vi "VA CoAP - Message - DECODE.vi"(0 "CoAP Message":string) -> (4 "CoAP Message Decoded":T1 {"Type" items=["CONfimable", "NON-confirmable", "ACKnowledgement", "ReSeT"]}, 8 "CoAP Message":u8[](array[numeric]), 10 "Valid?":bool, 15 "Format Error?":bool)   [LabVIEW 2020]
uses:
  data types/VA CoAP - Message.ctl
  data types/VA CoAP - Message - Type.ctl
  data types/VA CoAP - Message - Options.ctl
  data types/VA CoAP - Message - Options - 11 Uri-Path.ctl
panel:
  out "Paths":string[](array[string])
  out "Token Length":u8
  out "2nd LSB is 1?":bool
  out "1st LSB is 0?":bool
  out "Ate least 4 Bytes?":bool
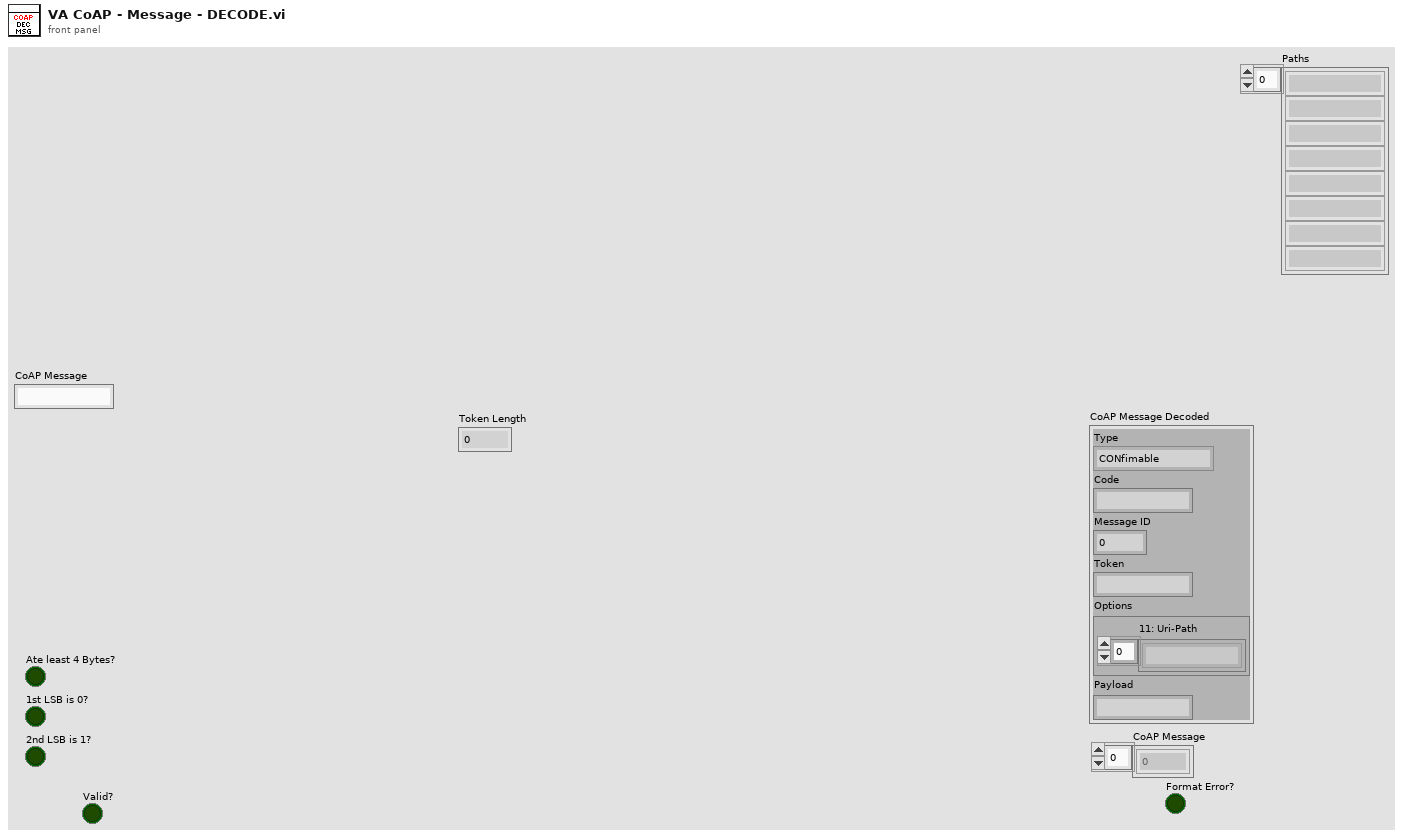
[diagram p1: front panel]
types:
  T1 = typedef "VA CoAP - Message.ctl" = cluster{"Type":T2, "Code":string, "Message ID":u16, "Token":string, "Options":T3, "Payload":string}
  T2 = typedef "VA CoAP - Message - Type.ctl" = u8
  T3 = typedef "VA CoAP - Message - Options.ctl" = cluster{"11: Uri-Path":T4}
  T4 = typedef "VA CoAP - Message - Options - 11 Uri-Path.ctl" = string[]
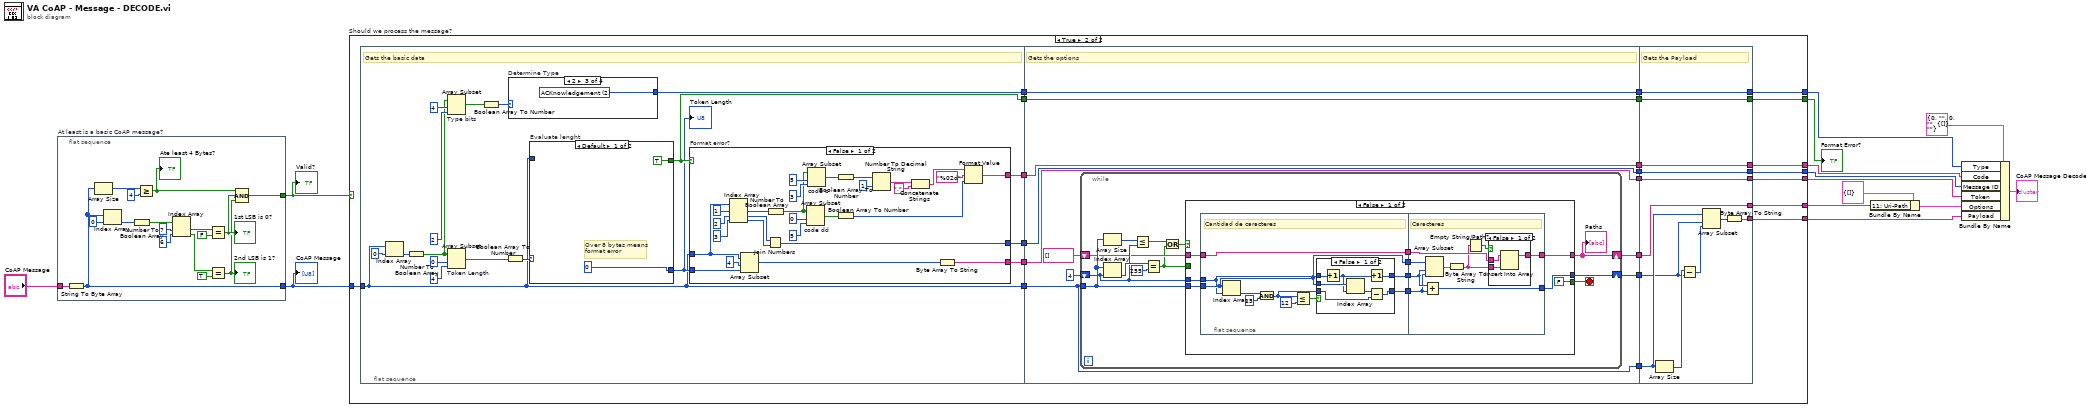
[diagram p0: block diagram]
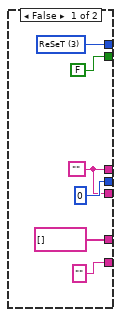
[diagram p2: hidden frame]
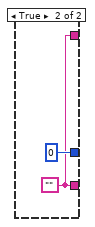
[diagram p3: hidden frame]
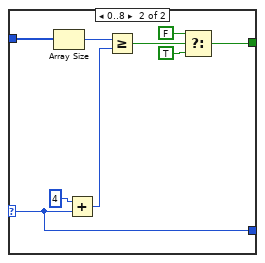
[diagram p4: hidden frame]
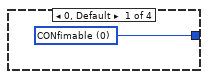
[diagram p5: hidden frame]
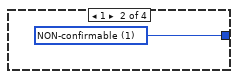
[diagram p6: hidden frame]
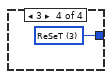
[diagram p7: hidden frame]
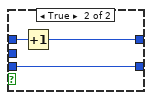
[diagram p8: hidden frame]
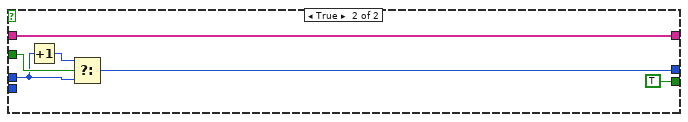
[diagram p10: hidden frame]
diagram:
  n1 = flat-sequence "At least is a basic CoAP message?" {
    tunnel: "CoAP Message" -> [w17]
    tunnel: [w16] -> w12
    tunnel: [w15] -> w5
    frame #0 {
      n2 = String To Byte Array(string=w17) -> (unsigned byte array=w15:u8[])
      n3 = Array Size(array=w15) -> (size(s)=w26:i32)
      n4 = Index Array(array=w15, index=0) -> (element=w30:u8)
      n5 = Number To Boolean Array(number=w30) -> (Boolean array=w29:bool[])
      n6 = Greater Or Equal?(x=w26, y=4) -> (x >= y?=w20:bool)
      "Ate least 4 Bytes?" <- w20
      n7 = Index Array(array=w29, index #1=7 ("index"), index #2=6 ("index")) -> (element #1=w24:bool, element #2=w21:bool)
      n8 = Equal?(x=w24, y=FALSE) -> (x = y?=w19:bool)
      "1st LSB is 0?" <- w19
      n9 = Equal?(x=w21, y=TRUE) -> (x = y?=w18:bool)
      "2nd LSB is 1?" <- w18
      n10 = Compound Arithmetic op=AND(w20, w19, w18) -> (w16:bool)
    }
  }
  n11 = case "Should we process the message?" shown="True" w12 {
    tunnel: w5 -> [_ w48]
    tunnel: [w37 w59] -> w10
    tunnel: [FALSE w58] -> w13
    tunnel: [w34 w57] -> w9
    tunnel: [u16 0 w56] -> w8
    tunnel: [w34 w55] -> w7
    tunnel: ["" ("string") w40] -> w4
    tunnel: [string[] [] w39] -> w1
    frame False {
      w34 = ""
      w37 = T2 3 items=["CONfimable", "NON-confirmable", "ACKnowledgement", "ReSeT"] ("Type 2")
    }
    frame True {
      n12 = flat-sequence {
        tunnel: w48 -> [w60]
        tunnel: [w71] -> w54
        tunnel: [w66] -> w53
        tunnel: [w65] -> w52
        tunnel: [w63] -> w51
        tunnel: [w62] -> w50
        tunnel: [w60] -> w49
        tunnel: w54 -> [w131]
        tunnel: w53 -> [w130]
        tunnel: w52 -> [w129]
        tunnel: w51 -> [w128]
        tunnel: w50 -> [w127]
        tunnel: w49 -> [w124]
        tunnel: [w131] -> w47
        tunnel: [w130] -> w46
        tunnel: [w129] -> w45
        tunnel: [w128] -> w44
        tunnel: [w127] -> w43
        tunnel: [w124] -> w42
        tunnel: [w123] -> w41
        tunnel: [w122] -> w38
        tunnel: [w200] -> w55
        tunnel: [w201] -> w56
        tunnel: [w202] -> w57
        tunnel: [w203] -> w58
        tunnel: [w204] -> w59
        tunnel: w47 -> [w204]
        tunnel: w46 -> [w203]
        tunnel: w45 -> [w202]
        tunnel: w44 -> [w201]
        tunnel: w43 -> [w200]
        tunnel: w42 -> [w196]
        tunnel: w41 -> [w195]
        tunnel: [w194] -> w40
        tunnel: [w193] -> w39
        tunnel: w38 -> [w193]
        frame #0 {
          # "Gets the basic data"
          n13 = Index Array(array=w60, index=0) -> (element=w76:u8)
          n14 = Number To Boolean Array(number=w76) -> (Boolean array=w64:bool[])
          n15 = Array Subset "Type bits"(array=w64, index=4, length=2) -> (w73:bool[])
          n16 = Array Subset "Token Length"(array=w64, index=0, length=4) -> (w68:bool[])
          n17 = Boolean Array To Number(Boolean array=w73) -> (number=w72:u32)
          n18 = Boolean Array To Number(Boolean array=w68) -> (number=w67:u32)
          n19 = case "Determine Type" shown="2" w72 {
            tunnel: [w118 w119 w120 w121] -> w71
            frame 0, Default {
              w118 = T2 0 items=["CONfimable", "NON-confirmable", "ACKnowledgement", "ReSeT"] ("Type 2")
            }
            frame 1 {
              w119 = T2 1 items=["CONfimable", "NON-confirmable", "ACKnowledgement", "ReSeT"] ("Type 2")
            }
            frame 2 {
              w120 = T2 2 items=["CONfimable", "NON-confirmable", "ACKnowledgement", "ReSeT"] ("Type 2")
            }
            frame 3 {
              w121 = T2 3 items=["CONfimable", "NON-confirmable", "ACKnowledgement", "ReSeT"] ("Type 2")
            }
          }
          n20 = case "Evaluate lenght" shown="Default" w67 {
            selector: w67 -> [_ w113]
            tunnel: [TRUE w109] -> w66
            tunnel: [u32 0 w113] -> w61
            tunnel: w60 -> [_ w117]
            frame Default {
              # "Over 8 bytes means\nformat error"
            }
            frame 0..8 {
              n21 = Array Size(array=w117) -> (size(s)=w116:i32)
              n22 = Add(x=4 ("length"), y=w113) -> (x+y=w115:u32)
              n23 = Greater Or Equal?(x=w116, y=w115) -> (x >= y?=w112:bool)
              n24 = Select(t=FALSE, s=w112, f=TRUE) -> (s? t:f=w109:bool)
            }
          }
          "Token Length" <- w61
          n25 = case "Format error?" shown="False" w66 {
            tunnel: w60 -> [w82 _]
            tunnel: [w88 w105] -> w65
            tunnel: [w83 u16 0] -> w63
            tunnel: w61 -> [w80 _]
            tunnel: [w78 w105] -> w62
            frame False {
              n26 = Index Array(array=w82, index #1=1 ("index"), index #2=2 ("index"), index #3=3 ("index")) -> (element #1=w103:u8, element #2=w85:u8, element #3=w84:u8)
              n27 = Array Subset(array=w82, index=4, length=w80) -> (w79:u8[])
              n28 = Join Numbers(hi=w85, lo=w84) -> ((hi.lo)=w83:u16)
              n29 = Number To Boolean Array(number=w103) -> (Boolean array=w100:bool[])
              n30 = Array Subset "code dd"(array=w100, index=0, length=5) -> (w96:bool[])
              n31 = Array Subset "code c"(array=w100, index=5, length=3) -> (w97:bool[])
              n32 = Boolean Array To Number(Boolean array=w97) -> (number=w95:u32)
              n33 = Boolean Array To Number(Boolean array=w96) -> (number=w90:u32)
              n34 = Number To Decimal String(number=w95, width (-)=i16 1) -> (decimal integer string=w93:string)
              n35 = Concatenate Strings(w93, "." ("string")) -> (w89:string)
              n36 = Byte Array To String(unsigned byte array=w79) -> (string=w78:string)
              n37 = Format Value(string ("")=w89, format string="%02d", value (0)=w90) -> (output string=w88:string)
            }
            frame True {
              w105 = ""
            }
          }
        }
        frame #1 {
          # "Gets the options"
          n38 = while {
            tunnel: w124 -> [w139]
            shift-right: [w137] -> w123
            shift-left: 4 ("index") -> [w138]
            shift-right: [w133] -> w122
            shift-left: string[] [] -> [w134]
            stop <- w135 stop-if-true
            n39 = Array Size(array=w139) -> (size(s)=w140:i32)
            n40 = Index Array(array=w139, index=w138) -> (element=w141:u8)
            n41 = Less Or Equal?(x=w140, y=w138) -> (x <= y?=w143:bool)
            n42 = Equal?(x=w141, y=u8 255) -> (x = y?=w132:bool)
            n43 = Or(x=w143, y=w132) -> (x .or. y?=w136:bool)
            n44 = case shown="False" w136 {
              tunnel: w139 -> [w150 _]
              tunnel: w138 -> [w149 w187]
              tunnel: [w148 w189] -> w137
              tunnel: [FALSE TRUE] -> w135
              tunnel: w134 -> [w145 w191]
              tunnel: [w144 w191] -> w133
              tunnel: w132 -> [_ w190]
              frame False {
                n45 = flat-sequence {
                  tunnel: w150 -> [w156]
                  tunnel: [w156] -> w153
                  tunnel: [w159] -> w152
                  tunnel: [w158] -> w151
                  tunnel: w149 -> [w155]
                  tunnel: [w154] -> w146
                  tunnel: w145 -> [w154]
                  tunnel: w153 -> [w179]
                  tunnel: w152 -> [w181]
                  tunnel: w151 -> [w180]
                  tunnel: [w178] -> w148
                  tunnel: w146 -> [w177]
                  tunnel: [w176] -> w144
                  frame #0 {
                    # "Cantidad de caracteres"
                    n46 = Index Array(array=w156, index=w155) -> (element=w162:u8)
                    n47 = And(x=w162, y=u8 15 ("index")) -> (x .and. y?=w157:u8)
                    n48 = Less Or Equal?(x=w157, y=u8 12) -> (x <= y?=w160:bool)
                    n49 = case shown="False" w160 {
                      tunnel: [w165 w172] -> w159
                      tunnel: [w167 w173] -> w158
                      tunnel: w157 -> [w168 w173]
                      tunnel: w156 -> [w170 _]
                      tunnel: w155 -> [w166 w171]
                      frame False {
                        n50 = Increment(x=w166) -> (x+1=w164:i32)
                        n51 = Index Array(array=w170, index=w164) -> (element=w169:u8)
                        n52 = Increment(x=w164) -> (x+1=w165:i32)
                        n53 = Subtract(x=w169, y=w168) -> (x-y=w167:u8)
                      }
                      frame True {
                        n54 = Increment(x=w171) -> (x+1=w172:i32)
                      }
                    }
                  }
                  frame #1 {
                    # "Caracteres"
                    n55 = Add(x=w181, y=w180) -> (x+y=w178:i32)
                    n56 = Array Subset(array=w179, index=w181, length=w180) -> (w182:u8[])
                    n57 = Byte Array To String(unsigned byte array=w182) -> (string=w175:string)
                    n58 = Empty String/Path?(string/path=w175) -> (empty?=w174:bool)
                    n59 = case shown="False" w174 {
                      tunnel: w177 -> [w185 w186]
                      tunnel: w175 -> [w184 _]
                      tunnel: [w183 w186] -> w176
                      frame False {
                        n60 = Insert Into Array(array=w185, new element=w184) -> (w183:string[])  [unwired: 1 in]
                      }
                      frame True {
                      }
                    }
                  }
                }
              }
              frame True {
                n61 = Increment(x=w187) -> (x+1=w188:i32)
                n62 = Select(t=w188, s=w190, f=w187) -> (s? t:f=w189:i32)
              }
            }
            "Paths" <- w133
          }
        }
        frame #2 {
          # "Gets the Payload"
          n63 = Array Size(array=w196) -> (size(s)=w199:i32)
          n64 = Subtract(x=w199, y=w195) -> (x-y=w198:i32)
          n65 = Array Subset(array=w196, index=w195, length=w198) -> (w197:u8[])
          n66 = Byte Array To String(unsigned byte array=w197) -> (string=w194:string)
        }
      }
    }
  }
  "Format Error?" <- w13
  n67 = Bundle By Name(cluster=T3 {"11: Uri-Path"=[]} ("Options"), "11: Uri-Path"=w1) -> (w2:T3)
  n68 = Bundle By Name(cluster=T1 {"Type"=0, "Code"="", "Message ID"=0, "Token"="", "Options"={"11: Uri-Path"=[]}, "Payload"=""} ("CoAP Message Basic Data"), "Type"=w10, "Code"=w9, "Message ID"=w8, "Token"=w7, "Options"=w2, "Payload"=w4) -> (→"CoAP Message Decoded":T1)
  "Valid?" <- w12
  "CoAP Message" <- w5
